vi "RW Tachometer TM.vi"(6 "low time":dbl=0.01 format="%.6f", 7 "high time":dbl=0.01 format="%.6f", 9 "Counter to Output with":tag="Dev1/ctr0") -> (0 "CO.CtrTimebaseSrc":tag, 1 "CO.Pulse.LowTime":dbl, 2 "CO.Pulse.HighTime":dbl, 3 "CO.Pulse.Term":tag, 4 "task done?":bool)   [LabVIEW 2019, in "SubVIs.lvlib" / "Tachometer VI.lvlib"]
uses:
  <vilib>/Utility/error.llb/DialogType.ctl
  <vilib>/DAQmx/create/channels.llb/DAQmx Create Channel (CO-Pulse Generation-Time).vi
  <vilib>/DAQmx/configure/timing.llb/DAQmx Timing (Implicit).vi
  Tachometer VI.lvlib
  <resource>/objmgr/daqmx.rc
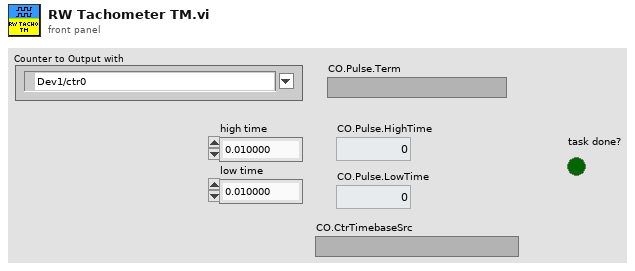
[diagram p1: front panel]
types:
  T1 = typedef "DialogType.ctl" = u16
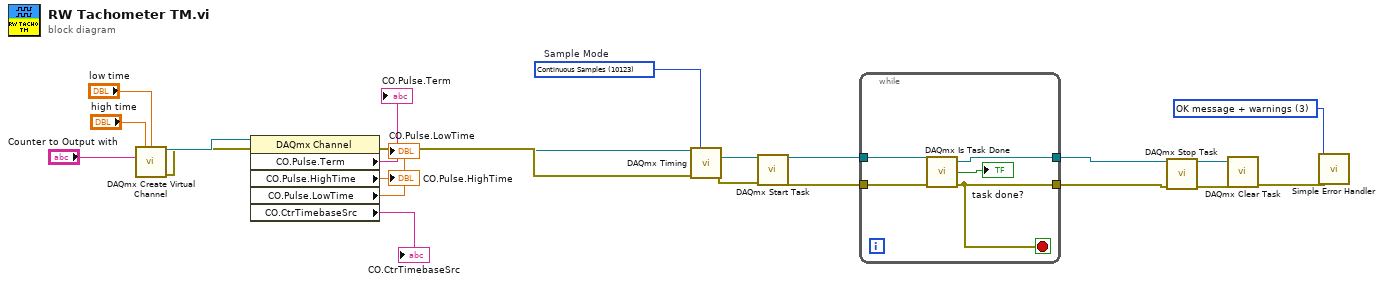
[diagram p0: block diagram]
diagram:
  w1 = T1 3 items=["no dialog", "OK message", "continue or stop message", "OK message + warnings", "continue/stop + warnings"] ("type of dialog (OK msg:1)")
  w22 = 10123 items=["Finite Samples"=10178, "Continuous Samples"=10123, "Hardware Timed Single Point"=12522]  # Sample Mode
  n1 = call-poly <vilib>:"DAQmx Create Virtual Channel.vi"("high time"="high time", "low time"="low time", "counter"="Counter to Output with") -> ("task out"=w20:refnum<k21>, "error out"=w19:errorcluster)  [unwired: 11 in]
  n2 = property class="DAQmx Channel"(reference=w20, error in=w19) -> (reference out=w17:refnum<k21>, error out=w18:errorcluster, "CO.Pulse.Term"=→"CO.Pulse.Term":tag, "CO.Pulse.HighTime"=→"CO.Pulse.HighTime":dbl, "CO.Pulse.LowTime"=→"CO.Pulse.LowTime":dbl, "CO.CtrTimebaseSrc"=→"CO.CtrTimebaseSrc":tag)
  n3 = call-poly <vilib>:"DAQmx Timing.vi"("task/channels in"=w17, "sample mode"=w22, "error in"=w18) -> ("task out"=w15:refnum<k21>, "error out"=w14:errorcluster)  [unwired: 11 in]
  n4 = call <vilib>:"DAQmx Start Task.vi"("task/channels in"=w15, "error in"=w14) -> ("task out"=w8:refnum<k21>, "error out"=w7:errorcluster)  [unwired: 12 in]
  n5 = while {
    tunnel: w8 -> [w27]
    tunnel: w7 -> [w26]
    tunnel: [w24] -> w6
    tunnel: [w23] -> w5
    stop <- w23 stop-if-true
    n6 = call <vilib>:"DAQmx Is Task Done.vi"("task/channels in"=w27, "error in"=w26) -> ("task out"=w24:refnum<k21>, "task done?"=→"task done?":bool, "error out"=w23:errorcluster)  [unwired: 11 in]
  }
  n7 = call <vilib>:"DAQmx Stop Task.vi"("task/channels in"=w6, "error in"=w5) -> ("task out"=w4:refnum<k21>, "error out"=w3:errorcluster)  [unwired: 12 in]
  n8 = call <vilib>:"DAQmx Clear Task.vi"("task in"=w4, "error in"=w3) -> ("error out"=w2:errorcluster)  [unwired: 13 in]
  n9 = call <vilib>:"Simple Error Handler.vi"("type of dialog (OK msg:1)"=w1, "error in (no error)"=w2) -> ()  [unwired: 3 in, 5 out]
